vi "fpga3.vi"() -> ()   [LabVIEW 2015]
uses:
  <vilib>/LabVIEW Targets/FPGA/RIO/nicrio_985x_controls.llb/CAN_IO_Frame Cluster.ctl
  <vilib>/LabVIEW Targets/FPGA/RIO/nicrio_985x_controls.llb/CAN_IO_Frame Type.ctl
  <vilib>/rvi/Emulation/niFpgaGetClockAttributes.vi
  <vilib>/rvi/Emulation/niFpgaSctlEmulationGetInTimedLoop.vi
  <vilib>/rvi/Emulation/niFpgaEmulationReportErrorSimple.vi
  <vilib>/rvi/eio/common/nirviEmuTemplateMethod_errors.vi
  <vilib>/rvi/Emulation/niFpgaCriticalErrorInLSC.vi
  <vilib>/eio/EIONode/EIONode.xnode
  <vilib>/eio/EIOMethodNode/EIOMethodNode.xnode
panel:
  out "Mod4/CAN1":T1={"timestamp high"=0, "timestamp low"=0, "identifier"=0, "type"=enum."Data Frame", "info A"=0, "info B"=0, "data length"=0, "data"=[0, 0, 0, 0, 0, 0, 0, 0]} {"identifier" format="%x"; "timestamp high" format="%08x"; "timestamp low" format="%08x"; "data" format="%.0x"}
  out "can0 error out1":errorcluster
  out "can0 error out":errorcluster
  out "m 760":u8[](array[numeric])
  out "m 729":u8[](array[numeric])
  out "m 728":u8[](array[numeric])
  out "m 727":u8[](array[numeric])
  out "m 726":u8[](array[numeric])
  out "m 725":u8[](array[numeric])
  out "m 724":u8[](array[numeric])
  out "m 723":u8[](array[numeric])
  out "m 722":u8[](array[numeric])
  out "m 721":u8[](array[numeric])
  out "m 720":u8[](array[numeric])
  out "m 711":u8[](array[numeric])
  out "m 710":u8[](array[numeric])
  out "m 700":u8[](array[numeric])
  out "Mod4/CAN0":T1={"timestamp high"=0, "timestamp low"=0, "identifier"=0, "type"=enum."Data Frame", "info A"=0, "info B"=0, "data length"=0, "data"=[0, 0, 0, 0, 0, 0, 0, 0]} {"identifier" format="%x"; "timestamp high" format="%08x"; "timestamp low" format="%08x"; "data" format="%.0x"}
  out "brk enc":u8
  in  "baud rate":i32(ring)=4 items=["300", "1200", "2400", "4800", "9600", "14400", "19200", "28800", "38400", "57600", "115200", "230400"]
  in  "B Pwm":u16
  in  "T Pwm":u16
  in  "S Pwm 1":u16
  in  "S Pwm 2":u16
  out "Auto":bool
  out "Run":bool
  in  "Solenoid":bool
  in  "Buzz":bool
  out "T Lim":bool
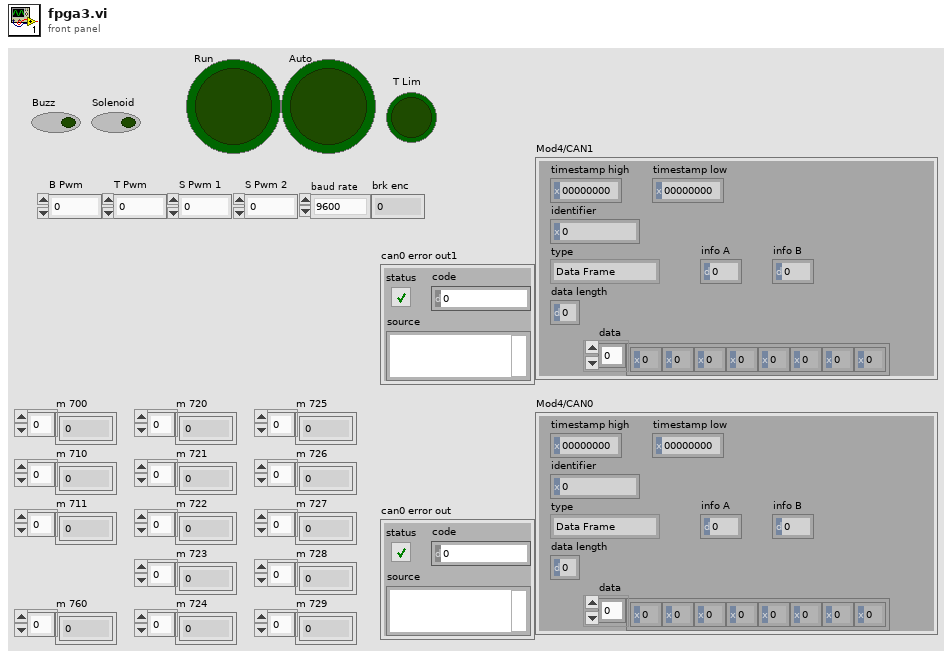
[diagram p1: front panel]
types:
  T1 = typedef "CAN_IO_Frame Cluster.ctl" = cluster{"timestamp high":u32, "timestamp low":u32, "identifier":u32, "type":T2, "info A":u8, "info B":u8, "data length":u8, "data":u8[]}
  T2 = typedef "CAN_IO_Frame Type.ctl" = enum8{"Data Frame", "Remote Frame", "(reserved)", "(reserved) ", "(reserved)  ", "(reserved)   ", "Bus Error", "Transceiver Fault"}
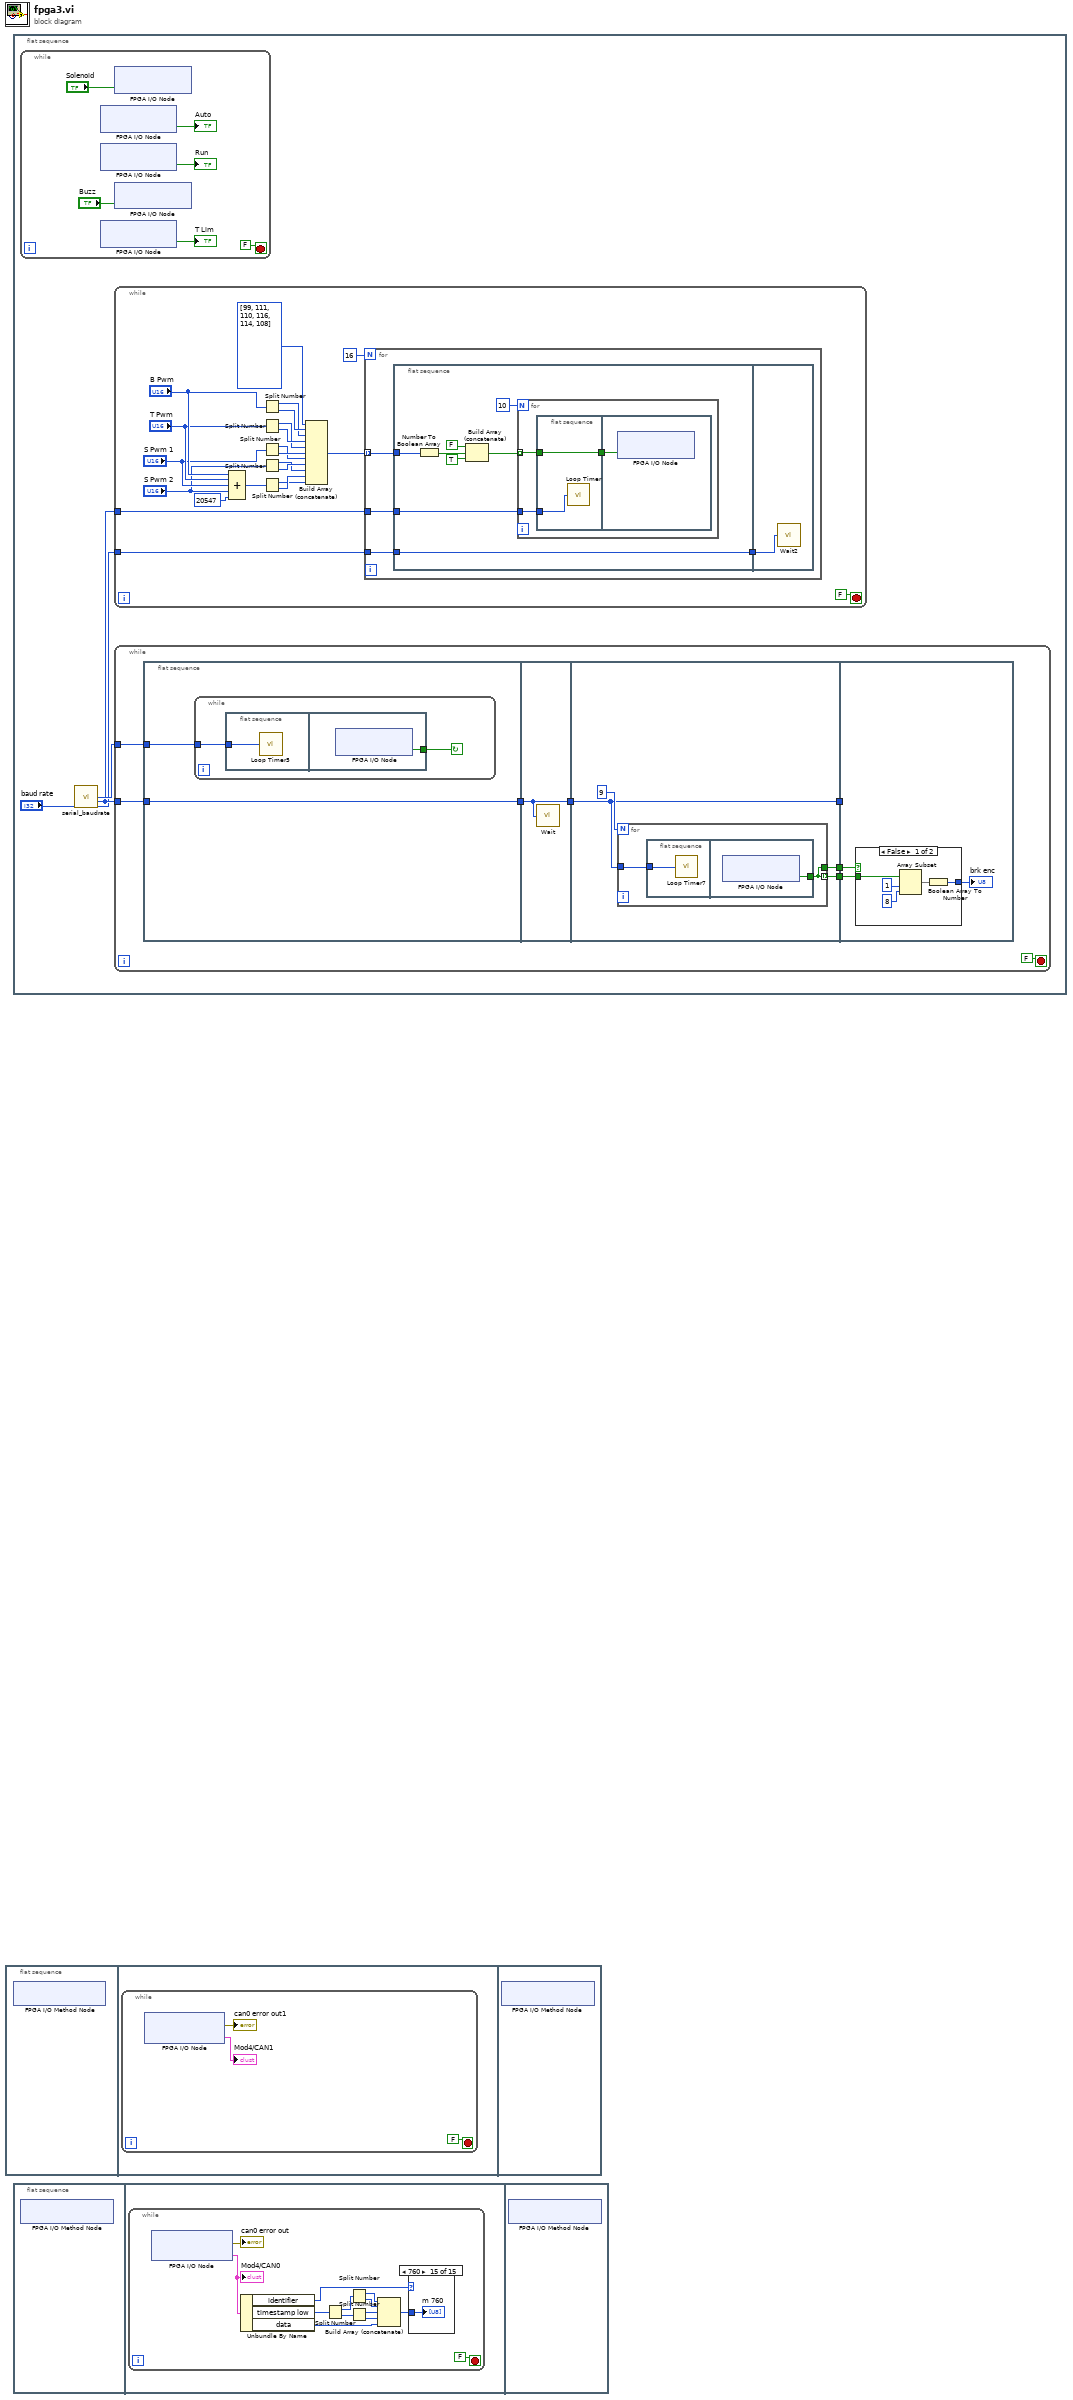
[diagram p0: block diagram]
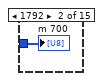
[diagram p3: hidden frame]
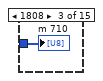
[diagram p4: hidden frame]
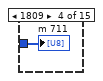
[diagram p5: hidden frame]
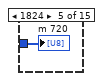
[diagram p6: hidden frame]
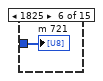
[diagram p7: hidden frame]
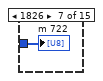
[diagram p8: hidden frame]
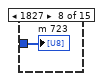
[diagram p9: hidden frame]
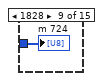
[diagram p10: hidden frame]
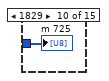
[diagram p11: hidden frame]
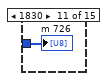
[diagram p12: hidden frame]
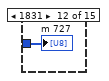
[diagram p13: hidden frame]
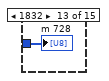
[diagram p14: hidden frame]
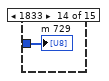
[diagram p15: hidden frame]
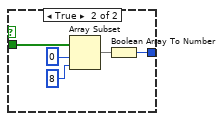
[diagram p16: hidden frame]
diagram:
  n1 = flat-sequence {
    frame #0 {
      n2 = xnode "FPGA I/O Method Node"() -> ()  [unwired: 1 in, 1 out]
    }
    frame #1 {
      n3 = while {
        stop <- FALSE stop-if-true
        n4 = xnode "FPGA I/O Node"() -> ("error out"=→"can0 error out1":errorcluster, "Mod4/CAN1"=→"Mod4/CAN1":T1)  [unwired: 2 in, 1 out]
      }
    }
    frame #2 {
      n5 = xnode "FPGA I/O Method Node"() -> ()  [unwired: 1 in, 1 out]
    }
  }
  n6 = flat-sequence {
    frame #0 {
      n7 = while {
        stop <- FALSE stop-if-true
        n8 = xnode "FPGA I/O Node"() -> ("Mod3/DIO0"=→"Auto":bool)  [unwired: 1 in, 1 out]
        n9 = xnode "FPGA I/O Node"() -> ("Mod3/DIO3"=→"Run":bool)  [unwired: 1 in, 1 out]
        n10 = xnode "FPGA I/O Node"() -> ("Mod3/DIO2"=→"T Lim":bool)  [unwired: 1 in, 1 out]
        n11 = xnode "FPGA I/O Node"("Mod3/DIO4"="Solenoid") -> ()  [unwired: 1 in, 1 out]
        n12 = xnode "FPGA I/O Node"("Mod3/DIO5"="Buzz") -> ()  [unwired: 1 in, 1 out]
      }
      n13 = call "serial_baudrate.vi"("baud rate"="baud rate") -> ("tick/2 every bit"=w6:u32, "tick every bit"=w5:u32, "tick after stop bit"=w4:u32)  [unwired: 12 in]
      n14 = while {
        tunnel: w5 -> [w9]
        tunnel: w4 -> [w8]
        stop <- FALSE stop-if-true
        n15 = Compound Arithmetic op=ADD("B Pwm", "T Pwm", "S Pwm 1", "S Pwm 2", u16 20547 ("value")) -> (w14:u16)
        n16 = Split Number(x="B Pwm") -> (hi(x)=w27:u8, lo(x)=w28:u8)
        n17 = Split Number(x="T Pwm") -> (hi(x)=w25:u8, lo(x)=w26:u8)
        n18 = Split Number(x="S Pwm 1") -> (hi(x)=w23:u8, lo(x)=w24:u8)
        n19 = Split Number(x="S Pwm 2") -> (hi(x)=w21:u8, lo(x)=w22:u8)
        n20 = Split Number(x=w14) -> (hi(x)=w12:u8, lo(x)=w13:u8)
        n21 = Build Array (concatenate)(u8[] [99, 111, 110, 116, 114, 108] ("header"), w28, w27, w26, w25, w24, w23, w22, w21, w13, w12) -> (w11:u8[])
        n22 = for {
          N: 16 -> [_]
          tunnel: w11 -> [w33] mode=indexing
          tunnel: w9 -> [w32]
          tunnel: w8 -> [w31]
          n23 = flat-sequence {
            tunnel: w33 -> [w41]
            tunnel: w32 -> [w40]
            tunnel: w31 -> [w34]
            tunnel: [w34] -> w30
            tunnel: w30 -> [w48]
            frame #0 {
              n24 = Number To Boolean Array(number=w41) -> (Boolean array=w39:bool[])
              n25 = Build Array (concatenate)(FALSE, w39, TRUE) -> (w36:bool[])
              n26 = for {
                N: 10 -> [_]
                tunnel: w36 -> [w43] mode=indexing
                tunnel: w40 -> [w42]
                n27 = flat-sequence {
                  tunnel: [w46] -> w44
                  tunnel: w43 -> [w46]
                  tunnel: w42 -> [w45]
                  tunnel: w44 -> [w47]
                  frame #0 {
                    n28 = call "Loop Timer"("Count(Ticks)"=w45) -> ()  [unwired: 1 out]
                  }
                  frame #1 {
                    n29 = xnode "FPGA I/O Node"("Mod3/DIO6"=w47) -> ()  [unwired: 1 in, 1 out]
                  }
                }
              }
            }
            frame #1 {
              n30 = call "Wait2"("Count(Ticks)"=w48) -> ()  [unwired: 1 out]
            }
          }
        }
      }
      n31 = while {
        tunnel: w5 -> [w51]
        tunnel: w6 -> [w50]
        stop <- FALSE stop-if-true
        n32 = flat-sequence {
          tunnel: w50 -> [w58]
          tunnel: [w57] -> w56
          tunnel: w51 -> [w57]
          tunnel: w56 -> [w63]
          tunnel: [w63] -> w55
          tunnel: [w66] -> w54
          tunnel: [w65] -> w53
          tunnel: w55 -> [w64]
          tunnel: [w64] -> w52
          tunnel: w54 -> [w72]
          tunnel: w53 -> [w74]
          tunnel: w52 -> [_]
          frame #0 {
            n33 = while {
              tunnel: w58 -> [w59]
              stop <- w60 continue-if-true
              n34 = flat-sequence {
                tunnel: w59 -> [w61]
                tunnel: [w62] -> w60
                frame #0 {
                  n35 = call "Loop Timer5"("Count(Ticks)"=w61) -> ()  [unwired: 1 out]
                }
                frame #1 {
                  n36 = xnode "FPGA I/O Node"() -> ("Mod3/DIO1"=w62:bool)  [unwired: 1 in, 1 out]
                }
              }
            }
          }
          frame #1 {
            n37 = call "Wait"("Count(Ticks)"=w63) -> ()  [unwired: 1 out]
          }
          frame #2 {
            n38 = for {
              N: 9 -> [_]
              tunnel: [w69] -> w65 mode=indexing
              tunnel: [w69] -> w66
              tunnel: w64 -> [w68]
              n39 = flat-sequence {
                tunnel: w68 -> [w70]
                tunnel: [w71] -> w69
                frame #0 {
                  n40 = call "Loop Timer7"("Count(Ticks)"=w70) -> ()  [unwired: 1 out]
                }
                frame #1 {
                  n41 = xnode "FPGA I/O Node"() -> ("Mod3/DIO1"=w71:bool)  [unwired: 1 in, 1 out]
                }
              }
            }
          }
          frame #3 {
            n42 = case shown="False" w72 {
              tunnel: w74 -> [w76 w81]
              tunnel: [w77 w82] -> w73
              frame False {
                n43 = Array Subset(array=w76, index=1, length=8) -> (w75:bool[])
                n44 = Boolean Array To Number(Boolean array=w75) -> (number=w77:u8)
              }
              frame True {
                n45 = Array Subset(array=w81, index=0, length=8) -> (w80:bool[])
                n46 = Boolean Array To Number(Boolean array=w80) -> (number=w82:u8)
              }
            }
            "brk enc" <- w73
          }
        }
      }
    }
  }
  n47 = flat-sequence {
    frame #0 {
      n48 = xnode "FPGA I/O Method Node"() -> ()  [unwired: 1 in, 1 out]
    }
    frame #1 {
      n49 = while {
        stop <- FALSE stop-if-true
        n50 = xnode "FPGA I/O Node"() -> ("error out"=→"can0 error out":errorcluster, "Mod4/CAN0"=w102:T1)  [unwired: 2 in, 1 out]
        "Mod4/CAN0" <- w102
        n51 = Unbundle By Name(w102) -> ("identifier"=w101:u32, "timestamp low"=w100:u32, "data"=w93:u8[])
        n52 = Split Number(x=w100) -> (hi(x)=w99:u16, lo(x)=w98:u16)
        n53 = Split Number(x=w99) -> (hi(x)=w97:u8, lo(x)=w96:u8)
        n54 = Split Number(x=w98) -> (hi(x)=w95:u8, lo(x)=w94:u8)
        n55 = Build Array (concatenate)(w97, w96, w95, w94, w93) -> (w92:u8[])
        n56 = case shown="760" w101 {
          tunnel: w92 -> [_ w104 w105 w106 w107 w108 w109 w110 w111 w112 w113 w114 w115 w116 w117]
          frame 0, Default {
          }
          frame 1792 {
            "m 700" <- w104
          }
          frame 1808 {
            "m 710" <- w105
          }
          frame 1809 {
            "m 711" <- w106
          }
          frame 1824 {
            "m 720" <- w107
          }
          frame 1825 {
            "m 721" <- w108
          }
          frame 1826 {
            "m 722" <- w109
          }
          frame 1827 {
            "m 723" <- w110
          }
          frame 1828 {
            "m 724" <- w111
          }
          frame 1829 {
            "m 725" <- w112
          }
          frame 1830 {
            "m 726" <- w113
          }
          frame 1831 {
            "m 727" <- w114
          }
          frame 1832 {
            "m 728" <- w115
          }
          frame 1833 {
            "m 729" <- w116
          }
          frame 1888 {
            "m 760" <- w117
          }
        }
      }
    }
    frame #2 {
      n57 = xnode "FPGA I/O Method Node"() -> ()  [unwired: 1 in, 1 out]
    }
  }
